vi "FPGA myRIOMain_v6.vi"() -> ()   [LabVIEW 2019]
doc: "Main FPGA VI\nUse the bitfile generated by this VI in the real-time code.\n\nv5: 16-pt Moving Average filter in AI sample loop"
uses:
  TypeDefs/AO mode TabCtrl.ctl
  TypeDefs/SamplingModeEnum.ctl
  <vilib>/Platform/TimedLoop/XDataNode/timing_clust.ctl
  <vilib>/Platform/TimedLoop/XDataNode/nitl_modes.ctl
  <vilib>/Platform/TimedLoop/XDataNode/wakeup.ctl
  <vilib>/rvi/Emulation/niFpgaGetClockAttributes.vi
  <vilib>/rvi/Emulation/niFpgaSctlEmulationGetInTimedLoop.vi
  <vilib>/rvi/Emulation/niFpgaEmulationReportErrorSimple.vi
  <vilib>/rvi/eio/common/nirviEmuTemplateMethod_errors.vi
  <vilib>/rvi/Emulation/niFpgaEmulationIsFPGAContextNoSignature.vi
  <vilib>/rvi/errors/niFpgaSetErrorForExecOnDevCompSimple.vi
  <vilib>/rvi/eio/common/nirviEmuReportErrorAndStop.vi
  <vilib>/rvi/DataTransferAndStorage/Container/Common/niFpgaContainerGetUniqueNameForEmu.vi
  <vilib>/rvi/FIFO/Fifo_Resource/nirvififoEmulationSetSize.vi
  <vilib>/rvi/FIFO/Fifo_Resource/nirviFifoEmulationQueueMgr.vi
  <instcachedir>/0/nirviFifoEmulationQueueMgr_E5CAEC123FF24DC58D834DCA3CDAA9B5.lvgen/nirviFifoEmulationQueueMgr_E5CAEC123FF24DC58D834DCA3CDAA9B5_008.vi
  <vilib>/rvi/FIFO/Fifo_Resource/nirvififoEmulationDetermineInputValidOut.vi
  <vilib>/rvi/FIFO/Fifo_Resource/nirvififoEmulationCreateLock.vi
  <vilib>/rvi/Emulation/niFpgaProcessEmulError.vi
  <vilib>/rvi/FIFO/Fifo_Resource/nirvififoEmulationObtainLock.vi
  <vilib>/rvi/FIFO/Fifo_Resource/nirvififoEmulationReleaseLock.vi
  <vilib>/rvi/occurrence/nirviWaitOnOccurrenceBase.vi
  <vilib>/rvi/errors/nirviReportUnexpectedCaseInternalError.vi
  <vilib>/rvi/errors/nirviReportUnexpectedCaseInternalError (U32).vi
  <vilib>/rvi/Emulation/niFpgaCriticalErrorInLSC.vi
  <instcachedir>/0/nirviFifoEmulationQueueMgr_E5CAEC123FF24DC58D834DCA3CDAA9B5.lvgen/nirviFifoEmulationQueueMgr_E5CAEC123FF24DC58D834DCA3CDAA9B5_003.vi
  <vilib>/Utility/error.llb/Clear Errors.vi
  <vilib>/rvi/Memory/Memory_Emulation/niFpgaMemoryEmulationCacheClearOnFirstRun.vi
  <vilib>/rvi/Memory/Memory_Emulation/nirvimemoryEmulationManagerCache_MakeExclusive.vi
  <vilib>/rvi/Memory/Memory_Emulation/niFpgaMemoryEmulationValidateCache.vi
  <vilib>/rvi/Memory/Memory_Emulation/nirvimemoryEmulationManagerCache_InsertValue.vi
  <vilib>/rvi/Memory/Memory_Emulation/nirvimemoryEmulationManagerCache_ReleaseExclusive.vi
  <vilib>/rvi/Memory/Memory_Emulation/nirvimemoryEmulationManagerCache_GetValue.vi
  <vilib>/rvi/Memory/Memory_Emulation/nirvimemoryEmulationManagerCache_SetValue.vi
  <vilib>/rvi/Analysis/common/codeGenErrors/XNode/niFpgaXNodeCodeGenErrorHandle.vi
  <vilib>/eio/EIONode/EIONode.xnode
  <vilib>/rvi/DataTransferAndStorage/Container/XNode/niFpgaContainer.xnode
  <vilib>/rvi/FIFO/Fifo_Resource/nirvififoEmulationWrite.vi
  <vilib>/rvi/FIFO/Fifo_Resource/nirvififoEmulationRead.vi
  <vilib>/rvi/DataTransferAndStorage/Register/Emulation/niFpgaRegisterEmulation.vi
  <vilib>/rvi/Analysis/measure/butterworth/XNode/niFpgaButterworthFilter.xnode
  <vilib>/rvi/FXPMathLib/FxpMul/XNode/nifxpmath_Multiplier.xnode
  <vilib>/rvi/Analysis/measure/LMRsmpl/XNode/niFPGA Rational Resampler.xnode
  <vilib>/Platform/TimedLoop/XDataNode/XDataNode.xnode
  FPGA functions/FPGA functions.lvlib
  <vilib>/rvi/FXPMathLib/sim/FxpSim.dll
  <vilib>/Platform/TimedLoop/XDataNode/XDNodeRunTimeDep.lvlib
panel:
  out "AI M Loop time [ticks]":u32
  out "FPGA AI DMA\nOverflow?":bool
  in  "AI Process Time [ticks]":u32=120
  out "Sample Freq. \ntoo high?":bool
  out "Processing Loop time [ticks]":u32
  out "AI Process. Freq.\ntoo high?":bool
  in  "Scaled Butterworth Coeffs":i32[](array[numeric])=[-1036986264, 2110353124, 93741, -1058362983, 2131726043, 94691]
  in  "Sampling Mode":T1
  in  "AO mode":T2
  in  "AO Out [V]":fxp<+/-,18,5> format="%#.6g"
  in  "AO enable?":bool
  out "AI In [V]":fxp<+/-,25,5> format="%#.6g"
  out "FPGA AO DMA\nOverflow?":bool
  out "Int. Output":i16
  out "Raw Int. Input":fxp<+/-,20,12> format="%.8g"
  in  "Sample Time [ticks]":u32=120
  out "AO Loop time [ticks]":u32
  out "AI Loop time [ticks]":u32
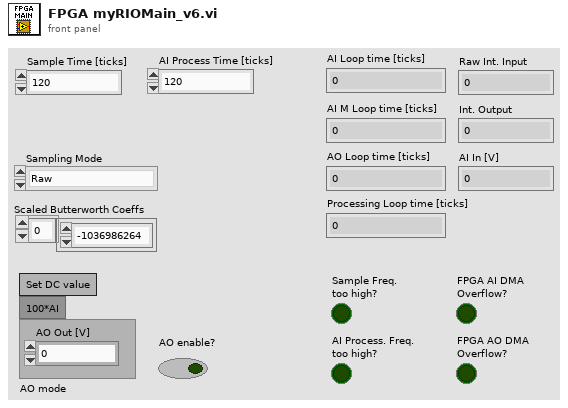
[diagram p1: front panel]
types:
  T1 = typedef "SamplingModeEnum.ctl" = enum16{"Raw", "4pt MA (AI)", "LPF (Proc.)", "4pt MA (AI) + LPF (Proc.)", "4pt MA (Proc.) + LPF (Proc.)"}
  T2 = typedef "AO mode TabCtrl.ctl" = enum32{"Set DC value", "100*AI"}
  T3 = typedef "XDNodeRunTimeDep.lvlib/timing_clust.ctl" = cluster{"Expected End [f-1]":u64, "Actual End [f-1]":u64, "Finished Late? [f-1]":bool, "Expected End [i-1]":u64, "Actual End [i-1]":u64, "Finished Late? [i-1]":bool, "Expected Start [i]":u64, "Actual Start [i]":u64, "Expected Start [f]":u64, "Actual Start [f]":u64, "Source Name":string, "Structure Name":string, "Period":i64, "Deadline":i64, "Offset":i64, "Start":i64, "Priority":i32, "Timeout":i32, "Mode":T4, "Wakeup Reason":T5, "Error":errorcluster, "Source Type":string, "Secondary Source Type":string, "Global End Time":u64, "Global Start Time":u64, "Frame Duration":u64, "Iteration Duration":u64, "Assigned CPU":i32, "I/O Scan Engine Mode":u32}
  T4 = typedef "XDNodeRunTimeDep.lvlib/nitl_modes.ctl" = enum32{"No Change", "Process missed periods, maintain original phase", "Discard missed periods, maintain original phase", "Process missed periods, ignore original phase", "Discard missed periods, ignore original phase"}
  T5 = typedef "XDNodeRunTimeDep.lvlib/wakeup.ctl" = enum32{"Normal", "Aborted", "Asynchronous wakeup", "Timing source error", "Timed loop error", "Timeout"}
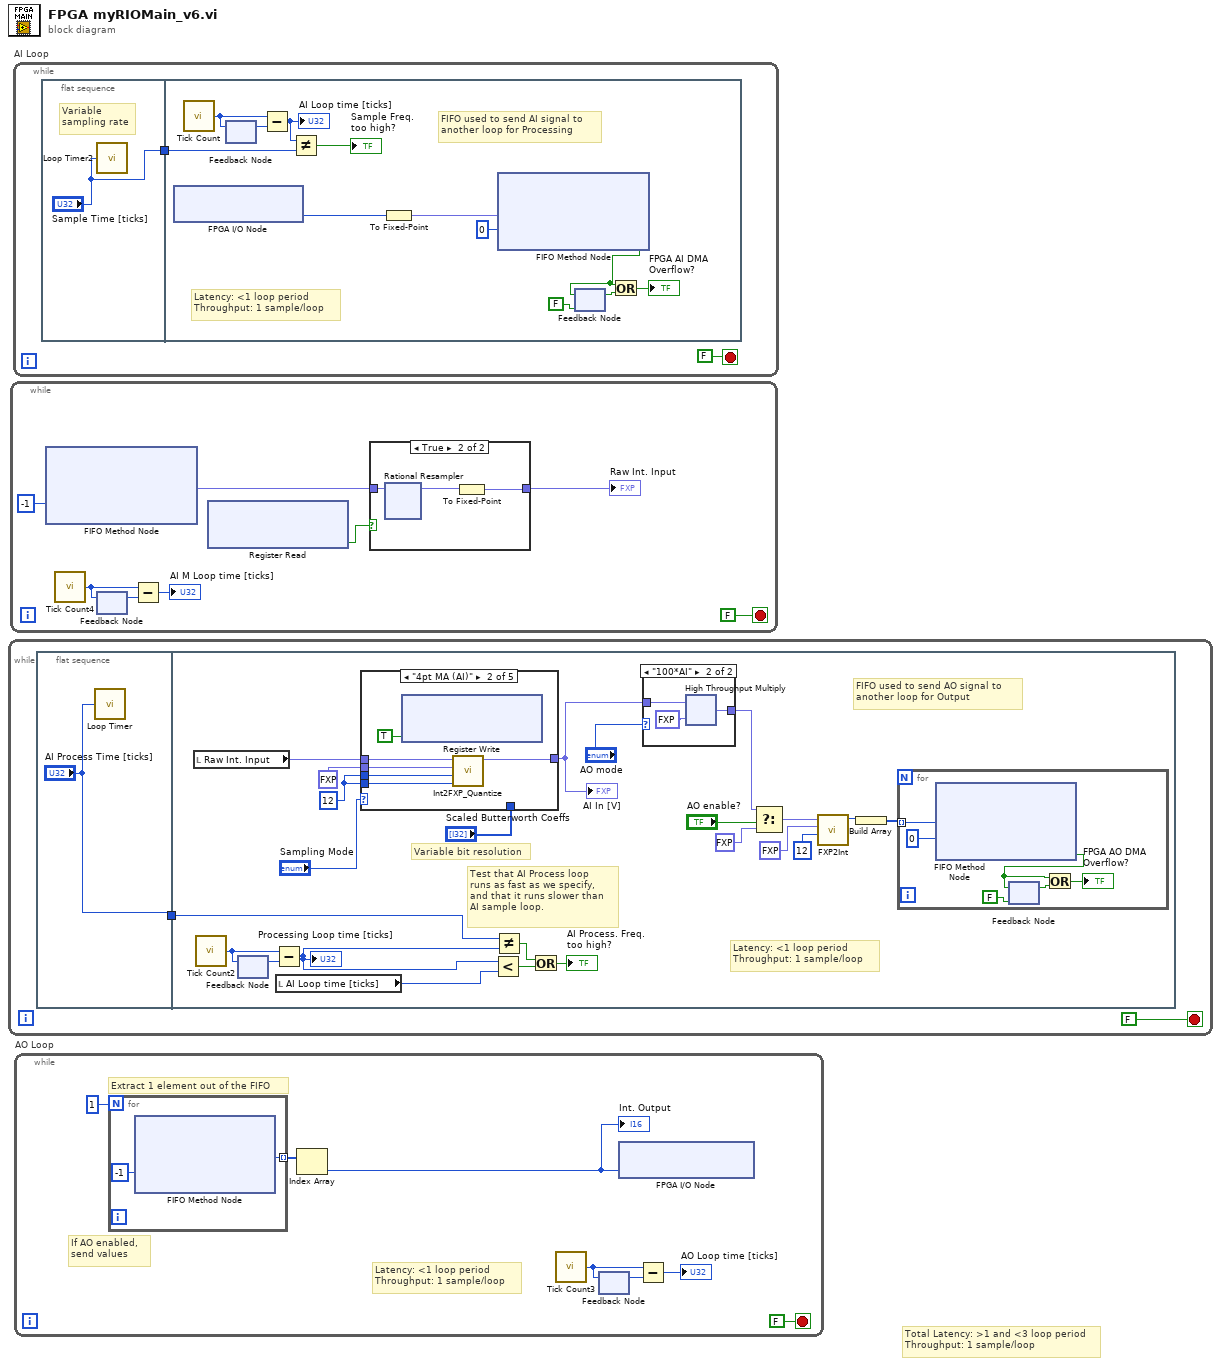
[diagram p0: block diagram]
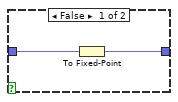
[diagram p2: hidden frame]
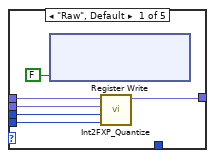
[diagram p3: hidden frame]
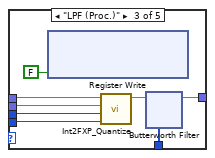
[diagram p4: hidden frame]
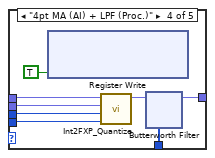
[diagram p5: hidden frame]
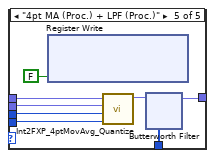
[diagram p6: hidden frame]
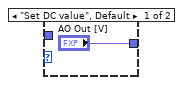
[diagram p7: hidden frame]
diagram:
  # "Total Latency: >1 and <3 loop period\nThroughput: 1 sample/loop"
  n1 = while {
    stop <- FALSE stop-if-true
    n2 = flat-sequence {
      tunnel: ["AI Process Time [ticks]"] -> w1
      tunnel: w1 -> [w6]
      frame #0 {
        n3 = call "Loop Timer"("Count(Ticks)"="AI Process Time [ticks]") -> ()  [unwired: 1 out]
      }
      frame #1 {
        w4 = i8 12 ("Input Bit resolution")
        # "Test that AI Process loop\nruns as fast as we specify,\nand that it runs slower than \nAI sample loop."
        # "Variable bit resolution"
        # "Latency: <1 loop period\nThroughput: 1 sample/loop"
        # "FIFO used to send AO signal to \nanother loop for Output"
        n4 = local read "Raw Int. Input"() -> (w11:fxp<+/-,20,12>)
        n5 = call "Tick Count2"() -> ("Tick Count(Ticks)"=w13:u32)
        n6 = feedback #1() -> (w12:u32)  [unwired: 1 in]
        n7 = feedback-in #1(w13) -> ()
        n8 = Subtract(x=w13, y=w12) -> (x-y=w5:u32)
        "Processing Loop time [ticks]" <- w5
        n9 = local read "AI Loop time [ticks]"() -> (w10:u32)
        n10 = case shown="\"4pt MA (AI)\"" "Sampling Mode" {
          tunnel: w4 -> [w32 w38 w43 w59 w77]
          tunnel: fxp<+,8,4> 10.0 ("Multiplier") -> [w31 w37 w44 w60 w78]
          tunnel: w4 -> [w30 w36 w42 w58 w76]
          tunnel: "Scaled Butterworth Coeffs" -> [_ _ w45 w61 w74]
          tunnel: [w29 w35 w41 w57 w73] -> w14
          tunnel: w11 -> [w28 w34 w40 w56 w72]
          frame "Raw", Default {
            n11 = xnode ("Register Write")("Data"=FALSE) -> ()  [unwired: 1 in, 1 out]
            n12 = call "Int2FXP_Quantize.vi"("Output Bit resolution"=w30, "Input Bit resolution"=w32, "Multiplier"=w31, "Input (Int)"=w28) -> ("Output (FXP)"=w29:fxp<+/-,25,5>)  [unwired: 7 in]
          }
          frame "4pt MA (AI)" {
            n13 = xnode ("Register Write")("Data"=TRUE) -> ()  [unwired: 1 in, 1 out]
            n14 = call "Int2FXP_Quantize.vi"("Output Bit resolution"=w36, "Input Bit resolution"=w38, "Multiplier"=w37, "Input (Int)"=w34) -> ("Output (FXP)"=w35:fxp<+/-,25,5>)  [unwired: 7 in]
          }
          frame "LPF (Proc.)" {
            n15 = xnode ("Register Write")("Data"=FALSE) -> ()  [unwired: 1 in, 1 out]
            n16 = call "Int2FXP_Quantize.vi"("Output Bit resolution"=w42, "Input Bit resolution"=w43, "Multiplier"=w44, "Input (Int)"=w40) -> ("Output (FXP)"=w46:fxp<+/-,25,5>)  [unwired: 7 in]
            n17 = xnode "Butterworth Filter"("input data"=w46, "scaled coefficients"=w45) -> ("output data"=w41:fxp<+/-,25,5>)  [unwired: 1 in]
          }
          frame "4pt MA (AI) + LPF (Proc.)" {
            n18 = xnode ("Register Write")("Data"=TRUE) -> ()  [unwired: 1 in, 1 out]
            n19 = call "Int2FXP_Quantize.vi"("Output Bit resolution"=w58, "Input Bit resolution"=w59, "Multiplier"=w60, "Input (Int)"=w56) -> ("Output (FXP)"=w62:fxp<+/-,25,5>)  [unwired: 7 in]
            n20 = xnode "Butterworth Filter"("input data"=w62, "scaled coefficients"=w61) -> ("output data"=w57:fxp<+/-,25,5>)  [unwired: 1 in]
          }
          frame "4pt MA (Proc.) + LPF (Proc.)" {
            n21 = xnode ("Register Write")("Data"=FALSE) -> ()  [unwired: 1 in, 1 out]
            n22 = call "Int2FXP_4ptMovAvg_Quantize.vi"("Output Bit resolution"=w76, "Input Bit resolution"=w77, "Multiplier"=w78, "Input (Int)"=w72) -> ("Output (FXP)"=w75:fxp<+/-,25,5>)  [unwired: 7 in]
            n23 = xnode "Butterworth Filter"("input data"=w75, "scaled coefficients"=w74) -> ("output data"=w73:fxp<+/-,25,5>)  [unwired: 1 in]
          }
        }
        "AI In [V]" <- w14
        n24 = Less?(x=w5, y=w10) -> (x < y?=w7:bool)
        n25 = Not Equal?(x=w6, y=w5) -> (x != y?=w8:bool)
        n26 = Or(x=w8, y=w7) -> (x .or. y?=→"AI Process. Freq.\ntoo high?":bool)
        n27 = case shown="\"100*AI\"" "AO mode" {
          tunnel: ["AO Out [V]" w88] -> w19
          tunnel: w14 -> [_ w90]
          frame "Set DC value", Default {
          }
          frame "100*AI" {
            n28 = xnode ("High Throughput Multiply")("x"=w90, "y"=fxp<+,5,7> 100.0) -> ("x*y"=w88:fxp<+/-,18,5>)
          }
        }
        n29 = Select(t=w19, s="AO enable?", f=fxp<+/-,18,5> 0.0) -> (s? t:f=w20:fxp<+/-,18,5>)
        n30 = call "FXP2Int.vi"("Output Bit resolution"=i8 12 ("Bit resolution"), "Multiplier"=fxp<+,18,-1> 0.10000038146972656, "Input (FXP)"=w20) -> ("Output (Int)"=w26:i16)  [unwired: 8 in]
        n31 = Build Array(w26) -> (w21:i16[])
        n32 = for {
          tunnel: w21 -> [w93] mode=indexing
          n33 = xnode ("FIFO Method Node")("Element"=w93, "Timeout"=0) -> ("Timed Out?"=w91:bool)  [unwired: 1 in, 1 out]
          n34 = feedback-in #2(w91) -> ()
          n35 = feedback #2(FALSE ("Timed Out?")) -> (w95:bool)
          n36 = Or(x=w91, y=w95) -> (x .or. y?=→"FPGA AO DMA\nOverflow?":bool)
        }
      }
    }
  }
  n37 = while {
    stop <- FALSE stop-if-true
    n38 = xnode ("FIFO Method Node")("Timeout"=-1) -> ("Element"=w99:fxp<+/-,16,12>)  [unwired: 1 in, 2 out]
    n39 = call "Tick Count4"() -> ("Tick Count(Ticks)"=w103:u32)
    n40 = feedback #3() -> (w102:u32)  [unwired: 1 in]
    n41 = feedback-in #3(w103) -> ()
    n42 = Subtract(x=w103, y=w102) -> (x-y=→"AI M Loop time [ticks]":u32)
    n43 = xnode ("Register Read")() -> ("Data"=w97:bool)  [unwired: 1 in, 1 out]
    n44 = case shown="True" w97 {
      tunnel: w99 -> [w105 w109]
      tunnel: [w106 w107] -> w98
      frame False {
        n45 = To Fixed-Point(number=w105) -> (fixed-point=w106:fxp<+/-,20,12>)  [unwired: 1 in]
      }
      frame True {
        n46 = xnode "Rational Resampler"("input data"=w109) -> ("output data"=w108:fxp<+/-,18,12>)  [unwired: 2 out]
        n47 = To Fixed-Point(number=w108) -> (fixed-point=w107:fxp<+/-,20,12>)  [unwired: 1 in]
      }
    }
    "Raw Int. Input" <- w98
  }
  n48 = while "AI Loop" {
    stop <- FALSE stop-if-true
    n49 = flat-sequence {
      tunnel: ["Sample Time [ticks]"] -> w144
      tunnel: w144 -> [w155]
      frame #0 {
        # "Variable\nsampling rate"
        n50 = call "Loop Timer2"("Count(Ticks)"="Sample Time [ticks]") -> ()  [unwired: 1 out]
      }
      frame #1 {
        # "FIFO used to send AI signal to \nanother loop for Processing"
        # "Latency: <1 loop period\nThroughput: 1 sample/loop"
        n51 = xnode "FPGA I/O Node"() -> ("ConnectorC/AI0"=w147:i16)  [unwired: 1 in, 1 out]
        n52 = call "Tick Count"() -> ("Tick Count(Ticks)"=w158:u32)
        n53 = feedback #4() -> (w157:u32)  [unwired: 1 in]
        n54 = feedback-in #4(w158) -> ()
        n55 = Subtract(x=w158, y=w157) -> (x-y=w156:u32)
        "AI Loop time [ticks]" <- w156
        n56 = Not Equal?(x=w156, y=w155) -> (x != y?=→"Sample Freq. \ntoo high?":bool)
        n57 = To Fixed-Point(number=w147) -> (fixed-point=w148:fxp<+/-,16,12>)  [unwired: 1 in]
        n58 = xnode ("FIFO Method Node")("Element"=w148, "Timeout"=0) -> ("Timed Out?"=w149:bool)  [unwired: 1 in, 1 out]
        n59 = feedback #5(FALSE ("Timed Out?")) -> (w151:bool)
        n60 = feedback-in #5(w149) -> ()
        n61 = Or(x=w149, y=w151) -> (x .or. y?=→"FPGA AI DMA\nOverflow?":bool)
      }
    }
  }
  n62 = while "AO Loop" {
    stop <- FALSE stop-if-true
    # "Latency: <1 loop period\nThroughput: 1 sample/loop"
    # "If AO enabled, \nsend values"
    # "Extract 1 element out of the FIFO"
    n63 = for {
      N: 1 -> [_]
      tunnel: [w167] -> w161 mode=indexing
      n64 = xnode ("FIFO Method Node")("Timeout"=-1) -> ("Element"=w167:i16)  [unwired: 1 in, 2 out]
    }
    n65 = Index Array(array=w161) -> (element=w159:i16)  [unwired: 1 in]
    "Int. Output" <- w159
    n66 = call "Tick Count3"() -> ("Tick Count(Ticks)"=w164:u32)
    n67 = feedback #6() -> (w163:u32)  [unwired: 1 in]
    n68 = feedback-in #6(w164) -> ()
    n69 = xnode "FPGA I/O Node"("ConnectorC/AO0"=w159) -> ()  [unwired: 1 in, 1 out]
    n70 = Subtract(x=w164, y=w163) -> (x-y=→"AO Loop time [ticks]":u32)
  }
